vi "M1T.vi"(8 "error in (no error)":errorcluster) -> (0 "error out":errorcluster, 3 "function return":dbl)   [LabVIEW 2014, in "MASTTCSGET.lvlib"]
doc: "primary mirror temperature\n\n\n\n__declspec (dllexport) float M1T();"
uses:
  MASTTCSGET.lvlib
  MASTTCSGET.dll
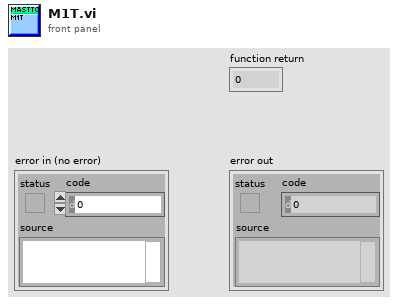
[diagram p1: front panel]
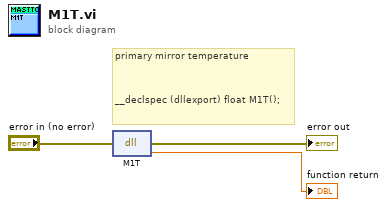
[diagram p0: block diagram]
diagram:
  # "primary mirror temperature\n\n\n\n__declspec (dllexport) float M1T();"
  n1 = dll-call lib="C:/Users/sanjay/Desktop/mast_controlsystem/MASTTCSGET.*" fn="M1T"(error in="error in (no error)") -> (error out=→"error out":errorcluster, →"function return":dbl)  [unwired: 2 in, 1 out]
